vi "calcbuffersv2.vi"(3 "refsize":i32) -> (0 "wfsize":i32, 1 "# of frames":i32)   [LabVIEW 2015]
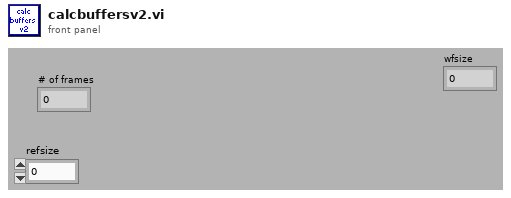
[diagram p1: front panel]
types:
  T1 = typedef "LVRectTypeDef.ctl" = cluster{"Left":i16, "Top":i16, "Right":i16, "Bottom":i16}
  T2 = cluster{"Xpixels":i32, "Vxminref":dbl, "Vxmaxref":dbl, "P":dbl, "Ypixels":i32, "Vyminref":dbl, "Vymaxref":dbl, "srate":sgl, "sAOxy":i32, "timeout":dbl, "type":string, "date":string, "time":string, "Colormap":u16, "Drawing Mode":u16, "Scanning Mode":u16, "square pixels":bool, "square matrix":bool, "Xpixels Img":i32, "Vx-min Img":dbl, "VX-max Img":dbl, "Ypixels Img":i32, "Vy-min Img":dbl, "Vy-max Img ":dbl, "Angle Img":dbl, "autoshutter":bool, "finite":bool, "cont":bool, "wavdet":bool, "measpoints":i32, "avpp":i32, "bufferAO":i32, "bufferAI":i32, "starttick":u32, "waveform":path, "Vx-ref":dbl, "Vy-ref":dbl, "refreshrate":dbl, "refreshbuffer":i32, "tt_cycles":i32, "motorref":refnum<k7>, "mirrorswitch":refnum<k7>, "sample mode":i32, "maxbufferAI":i32, "srateAODO":sgl, "bin":sgl, "Pel":sgl, "Angle draw":dbl, "srate Img":sgl, "ROIimg_plotbounds":T1, "auto OD":bool, "ODfilt":u16, "aAI":i32[], "aCI":i32[], "aAO":u32[], "aDO":u32[], "refwfsize":dbl, "Lifetime":bool, "Vz-Img":dbl, "Vz-ref":dbl, "Vz-reset":dbl, "AIoverride":bool, "aAS":u32[], "XYZstart":dbl[]}
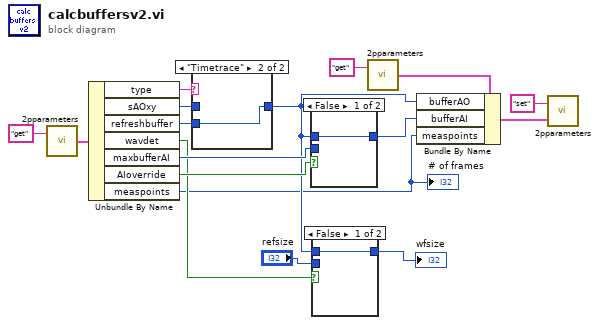
[diagram p0: block diagram]
diagram:
  n1 = call "2pparameters.vi"("command"="get") -> ("params out"=w9:T2)  [unwired: 1 in]
  n2 = Unbundle By Name(w9) -> ("type"=w2:string, "sAOxy"=w4:i32, "refreshbuffer"=w5:i32, "wavdet"=w10:bool, "maxbufferAI"=w16:i32, "AIoverride"=w15:bool, "measpoints"=w1:i32)
  "# of frames" <- w1
  n3 = case shown="\"Timetrace\"" w2 {
    tunnel: w5 -> [_ w19]
    tunnel: w4 -> [w18 _]
    tunnel: [w18 w19] -> w3
    frame "Lifetime (scan)", "X-Y-Z stack", "X-Y-t movie", Default {
    }
    frame "Timetrace" {
    }
  }
  n4 = case shown="False" w15 {
    tunnel: [w20 w21] -> w17
    tunnel: w16 -> [_ w21]
    tunnel: w3 -> [w20 _]
    frame False {
    }
    frame True {
    }
  }
  n5 = case shown="False" w10 {
    tunnel: w3 -> [w22 _]
    tunnel: [w22 w23] -> w6
    tunnel: "refsize" -> [_ w23]
    frame False {
    }
    frame True {
    }
  }
  "wfsize" <- w6
  n6 = call "2pparameters.vi"("command"="get") -> ("params out"=w11:T2)  [unwired: 1 in]
  n7 = Bundle By Name(cluster=w11, "bufferAO"=w3, "bufferAI"=w17, "measpoints"=w1) -> (w12:T2)
  n8 = call "2pparameters.vi"("Params in"=w12, "command"="set") -> ()  [unwired: 1 out]
